vi "GE5565 Set DMA Transfer Size.vi"(4 "error in (no error)":errorcluster, 6 "Transfer Size":u32, 7 "VMIC-5565":T1) -> (0 "error out":errorcluster, 3 "VMIC-5565":T1)   [LabVIEW 2019, in "RefMem DMA Engine.lvlib"]
uses:
  RefMem DMA Engine.lvlib
  <vilib>/Instr/_visa.llb/VISA Register Access Address Space.ctl
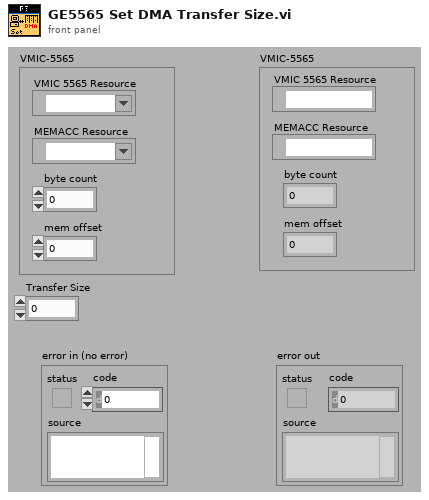
[diagram p1: front panel]
types:
  T1 = cluster{"VMIC 5565 Resource":refnum<visa-resource-name>, "MEMACC Resource":refnum<visa-resource-name>, "byte count":u32, "mem offset":u32}
  T2 = typedef "VISA Register Access Address Space.ctl" = u16
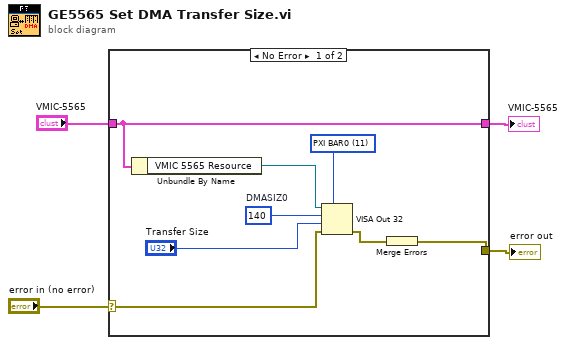
[diagram p0: block diagram]
diagram:
  n1 = case shown="No Error" "error in (no error)" {
    selector: "error in (no error)" -> [w10 w13]
    tunnel: "VMIC-5565" -> [w8 w14]
    tunnel: [w8 w14] -> w1
    tunnel: [w11 w13] -> w3
    frame No Error {
      w6 = u32 140  # DMASIZ0
      w7 = T2 11 items=["VXI/VME A16"=1, "VXI/VME A24"=2, "VXI/VME A32"=3, "VXI/VME A64"=4, "PXI Memory Allocations"=9, "PXI Configuration"=10, "PXI BAR0"=11, "PXI BAR1"=12, "PXI BAR2"=13, "PXI BAR3"=14, "PXI BAR4"=15, "PXI BAR5"=16] ("Address Space")
      n2 = Unbundle By Name(w8) -> ("VMIC 5565 Resource"=w9:refnum<visa-resource-name>)
      n3 = VISA Out 32(7:w7, 8:w10, 9:"Transfer Size", 10:w6, 11:w9) -> (0:w12:errorcluster)  [unwired: 1 out]
      n4 = Merge Errors(w12) -> (w11:errorcluster)
    }
    frame Error {
    }
  }
  "error out" <- w3
  "VMIC-5565" <- w1
